vi "getStatus.vi"(0 "HGF_Queue in":refnum<class "HGF_Queue.lvclass">, 2 "return elements? (F)":bool, 5 "error in (no error)":errorcluster) -> (10 "max queue size":i32, 11 "elements":refnum<class>[](array[class]), 12 "queue name":string, 13 "# elements in queue":i32, 14 "HGF_Queue out":refnum<class "HGF_Queue.lvclass">, 15 "# pending remove":i32, 16 "# pending insert":i32, 19 "error out":errorcluster)   [LabVIEW 2014, in "HGF_BaseClasses.lvlib" / "HGF_Queue.lvclass"]
doc: "Get queue status."
uses:
  HGF_Queue.lvclass
  HGF_Auxiliary/HGF_Auxiliary.lvlib
  HGF_Auxiliary/ErrorCode.ctl
  HGF_Auxiliary/Severity.ctl
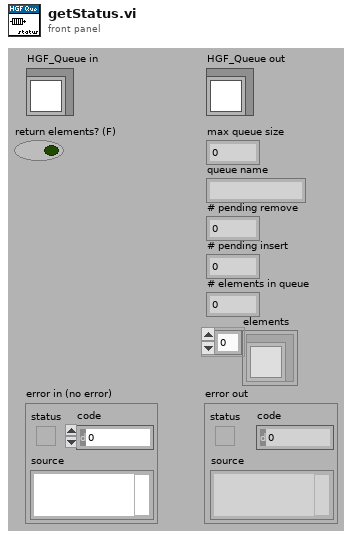
[diagram p1: front panel]
types:
  T1 = typedef "HGF_Auxiliary.lvlib/Severity.ctl" = enum16{"Info", "Warning", "Fault", "Error", "Fatal"}
  T2 = typedef "HGF_Auxiliary.lvlib/ErrorCode.ctl" = enum32{"No error", "Function not supported.", "This VI is for friends only.", "Reference object aready exisits.", "Parameter out of range.", "Not a rendezvous.", "Invalid notifier reference.", "Invalid queue reference.", "Self-Test not supported.", "Reset not supported.", "IDN query not supported.", "Error query not supported.", "Incorrect addressee.", "Object already exists.", "No class name specified", "Driver not supported", "Attribute is not writable"}
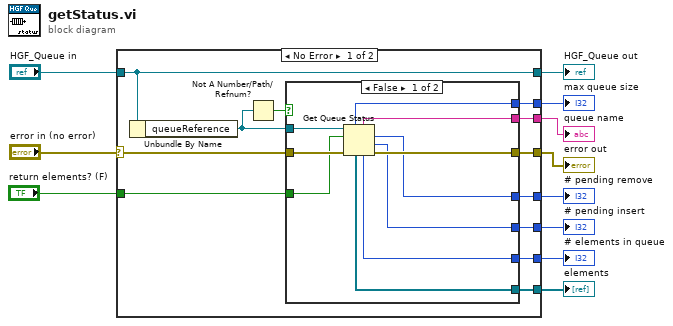
[diagram p0: block diagram]
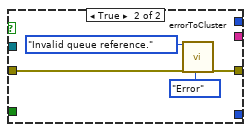
[diagram p2: hidden frame]
diagram:
  n1 = case shown="No Error" "error in (no error)" {
    selector: "error in (no error)" -> [w20 w39]
    tunnel: [w21 w39] -> w10
    tunnel: [w23 w38] -> w8
    tunnel: "HGF_Queue in" -> [w23 w38]
    tunnel: "return elements? (F)" -> [w18 _]
    tunnel: [w17 _] -> w6
    tunnel: [w16 _] -> w5
    tunnel: [w15 _] -> w4
    tunnel: [w14 _] -> w3
    tunnel: [w13 _] -> w2
    tunnel: [w12 _] -> w1
    frame No Error {
      n2 = Unbundle By Name(w23) -> ("queueReference"=w22:refnum<queue>)
      n3 = Not A Number/Path/Refnum?(number/path/refnum=w22) -> (NaN/Path/Refnum?=w19:bool)
      n4 = case shown="False" w19 {
        tunnel: w22 -> [w33 _]
        tunnel: [w32 w36] -> w21
        tunnel: w20 -> [w31 w37]
        tunnel: w18 -> [w30 _]
        tunnel: [w29 _] -> w17
        tunnel: [w28 _] -> w16
        tunnel: [w27 _] -> w15
        tunnel: [w26 _] -> w14
        tunnel: [w25 _] -> w13
        tunnel: [w24 _] -> w12
        frame False {
          n5 = Get Queue Status(queue=w33, return elements? (F)=w30, error in (no error)=w31) -> (queue name=w28:string, max queue size=w29:i32, # pending remove=w27:i32, # pending insert=w26:i32, error out=w32:errorcluster, # elements in queue=w25:i32, elements=w24:refnum<class>[])  [unwired: 1 out]
        }
        frame True {
          n6 = call "errorToCluster.vi"("error code"=ErrorCode."Invalid queue reference.", "error in (no error)"=w37, "severity (Error)"=Severity."Error") -> ("error out"=w36:errorcluster)  [unwired: 2 in, 14 out]
        }
      }
    }
    frame Error {
    }
  }
  "error out" <- w10
  "HGF_Queue out" <- w8
  "max queue size" <- w6
  "queue name" <- w5
  "elements" <- w1
  "# elements in queue" <- w2
  "# pending insert" <- w3
  "# pending remove" <- w4
